vi "Example.vi"() -> ()   [LabVIEW 2015]
uses:
  BufferConfig.ctl
  BufferLogging.lvlib
panel:
  out "snapshot":sgl[][](graph)
  in  "logging trigger":bool
  in  "stop":bool
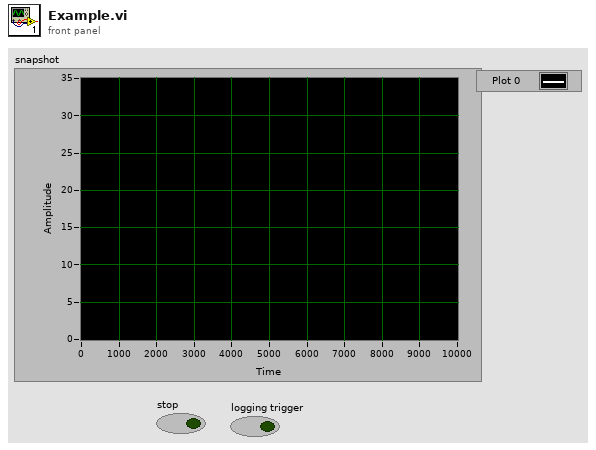
[diagram p1: front panel]
types:
  T1 = typedef "BufferLogging.lvlib/BufferConfig.ctl" = cluster{"Channels":string[], "pretriggerTime_sec":dbl, "posttriggerTime_sec":dbl, "BlockSizePerChannel":i32, "SampleRate_Hz":dbl, "decimation factor":i32, "logDirectory":path, "logPrefix":string, "max files":i32}
  T2 = typedef "BufferLogging.lvlib/Buffers.ctl" = cluster{"Channels":string[], "PosttriggerBuffer":refnum<queue>, "PretriggerBuffer":refnum<queue>, "BlockSizePerChannel":i32, " logging semaphore":T3, "Log refnum":refnum<k34>, "snapshotBuffer":refnum<data-value>, "logDirectory":path, "logPrefix":string, "decimation factor":i32, "max files":i32, "SampleRate":dbl}
  T3 = typedef "Semaphore RefNum" = refnum<k1>
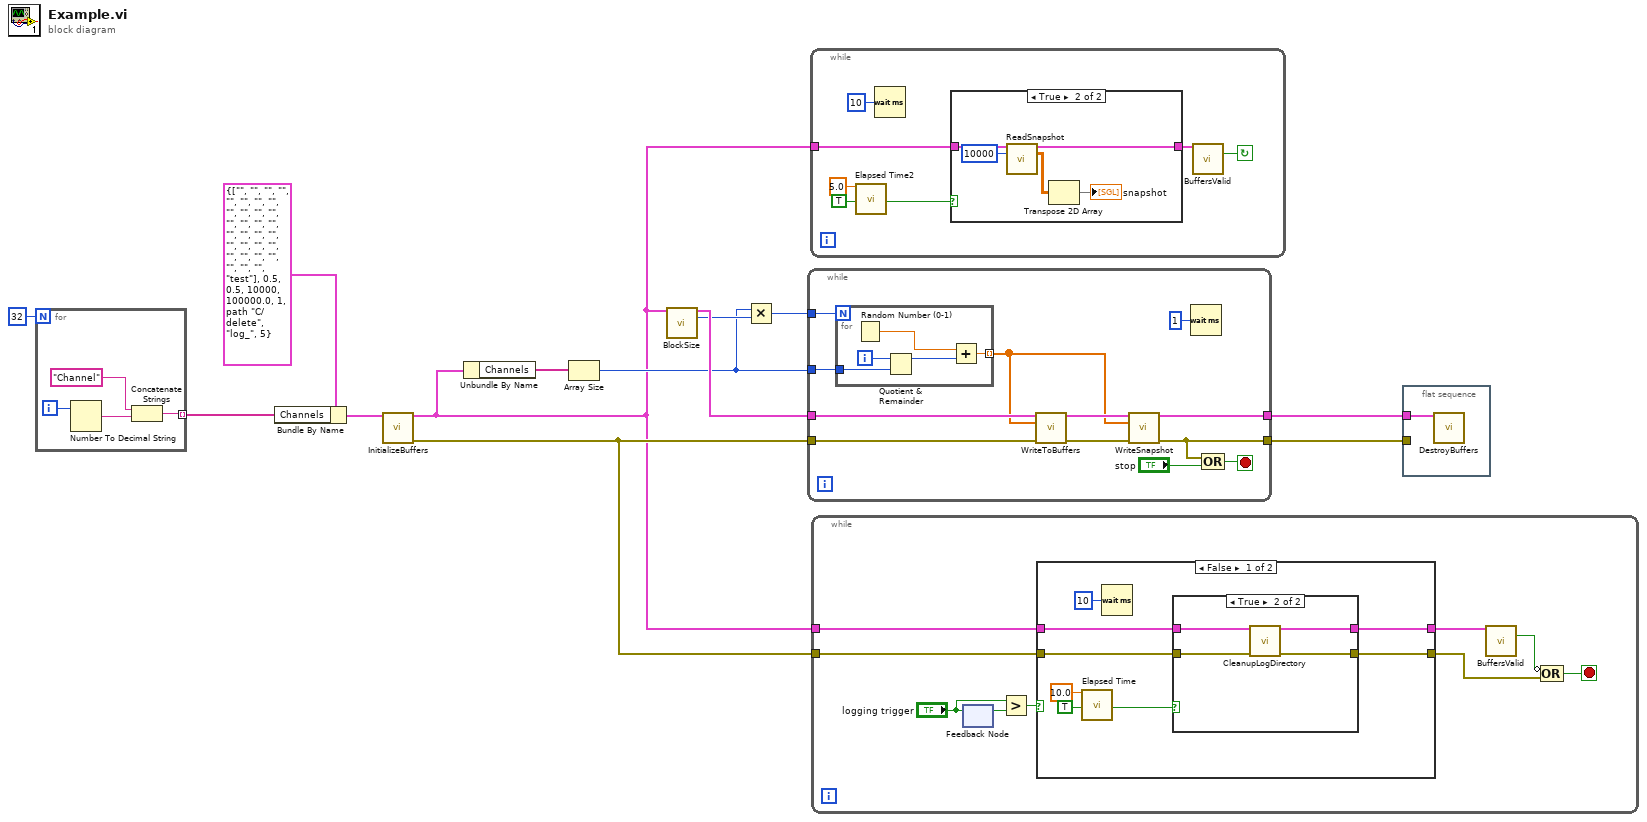
[diagram p0: block diagram]
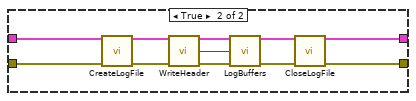
[diagram p4: hidden frame]
diagram:
  n1 = for {
    N: 32 -> [_]
    tunnel: [w14] -> w4 mode=indexing
    i -> [w17]
    n2 = Number To Decimal String(number=w17) -> (decimal integer string=w16:string)  [unwired: 1 in]
    n3 = Concatenate Strings("Channel", w16) -> (w14:string)
  }
  n4 = Bundle By Name(cluster=T1 {"Channels"=["", "", "", "", "", "", "", "", "", "", "", "", "", "", "", "", "", "", "", "", "", "", "", "", "", "", "", "", "", "", "", "test"], "pretriggerTime_sec"=0.5, "posttriggerTime_sec"=0.5, "BlockSizePerChannel"=10000, "SampleRate_Hz"=100000.0, "decimation factor"=1, "logDirectory"=path "C:/delete", "logPrefix"="log_", "max files"=5} ("BufferConfig"), "Channels"=w4) -> (w5:T1)
  n5 = call "InitializeBuffers.vi"("BufferConfig"=w5) -> ("Buffers"=w1:T2, "error out"=w3:errorcluster)  [unwired: 13 in]
  n6 = Unbundle By Name(w1) -> ("Channels"=w8:string[])
  n7 = Array Size(array=w8) -> (size(s)=w7:i32)
  n8 = call "BlockSize.vi"("BuffersIn"=w1) -> ("BuffersOut"=w12:T2, "BlockSize"=w10:i32)  [unwired: 13 in]
  n9 = Multiply(x=w7, y=w10) -> (x*y=w9:i32)
  n10 = while {
    tunnel: w12 -> [w29]
    tunnel: w3 -> [w28]
    tunnel: [w25] -> w13
    tunnel: w9 -> [w22]
    tunnel: [w20] -> w11
    tunnel: w7 -> [w18]
    stop <- w24 stop-if-true
    n11 = for {
      N: w22 -> [_]
      tunnel: [w33] -> w21 mode=indexing
      tunnel: w18 -> [w30]
      i -> [w32]
      n12 = Random Number (0-1)() -> (number: 0 to 1=w34:dbl)
      n13 = Quotient & Remainder(x=w32, y=w30) -> (x-y*floor(x/y)=w31:i32)  [unwired: 1 out]
      n14 = Add(x=w34, y=w31) -> (x+y=w33:dbl)
    }
    n15 = call "WriteToBuffers.vi"("Buffers in"=w29, "Data"=w21, "error in (no error)"=w28) -> ("Buffers out"=w27:T2, "error out"=w26:errorcluster)  [unwired: 11 in]
    n16 = call "WriteSnapshot.vi"("Buffers in"=w27, "Snapshot"=w21, "error in (no error)"=w26) -> ("Buffers out"=w25:T2, "error out"=w20:errorcluster)  [unwired: 11 in]
    n17 = Wait (ms)(milliseconds to wait=u32 1) -> ()  [unwired: 1 out]
    n18 = Compound Arithmetic op=OR(w20, "stop") -> (w24:bool)
  }
  n19 = while {
    tunnel: w1 -> [w41]
    stop <- w39 continue-if-true
    n20 = call "Elapsed Time2"("Time Target (s)"=5.0, "Auto Reset"=TRUE) -> ("Time has Elapsed"=w36:bool)  [unwired: 10 in, 7 out]
    n21 = Wait (ms)(milliseconds to wait=u32 10) -> ()  [unwired: 1 out]
    n22 = case shown="True" w36 {
      tunnel: w41 -> [w42 w47]
      tunnel: [w42 w46] -> w40
      frame False {
      }
      frame True {
        n23 = call "ReadSnapshot.vi"("Buffers in"=w47, "sizeOfBlock"=10000) -> ("Buffers out"=w46:T2, "snapshot"=w44:sgl[][])  [unwired: 11 in, 1 out]
        n24 = Transpose 2D Array(2D array=w44) -> (transposed array=→"snapshot":sgl[][])
      }
    }
    n25 = call "BuffersValid.vi"("Buffers in"=w40) -> ("valid"=w39:bool)  [unwired: 13 in, 1 out]
  }
  n26 = while {
    tunnel: w3 -> [w53]
    tunnel: w1 -> [w52]
    stop <- w50 stop-if-true
    n27 = feedback-in #1("logging trigger") -> ()
    n28 = feedback #1() -> (w55:bool)  [unwired: 1 in]
    n29 = Greater?(x="logging trigger", y=w55) -> (0:w54:bool)
    n30 = case shown="False" w54 {
      tunnel: w53 -> [w60 w81]
      tunnel: w52 -> [w58 w80]
      tunnel: [w57 w72] -> w51
      tunnel: [w59 w71] -> w48
      frame False {
        n31 = call "Elapsed Time"("Time Target (s)"=10.0, "Auto Reset"=TRUE) -> ("Time has Elapsed"=w61:bool)  [unwired: 10 in, 7 out]
        n32 = Wait (ms)(milliseconds to wait=u32 10) -> ()  [unwired: 1 out]
        n33 = case shown="True" w61 {
          tunnel: w60 -> [w66 w70]
          tunnel: [w66 w69] -> w59
          tunnel: w58 -> [w65 w68]
          tunnel: [w65 w67] -> w57
          frame False {
          }
          frame True {
            n34 = call "CleanupLogDirectory.vi"("BuffersIn"=w68, "error in"=w70) -> ("BuffersOut"=w67:T2, "error out"=w69:errorcluster)  [unwired: 12 in]
          }
        }
      }
      frame True {
        n35 = call "CreateLogFile.vi"("Buffers in"=w80, "error in (no error)"=w81) -> ("Buffers out"=w79:T2, "error out"=w78:errorcluster)  [unwired: 12 in]
        n36 = call "WriteHeader.vi"("Buffers in"=w79, "error in (no error)"=w78) -> ("Buffers out"=w77:T2, "numOfChannels"=w75:i32, "error out"=w76:errorcluster)  [unwired: 11 in]
        n37 = call "LogBuffers.vi"("Buffers in"=w77, "numOfChannels"=w75, "error in (no error)"=w76) -> ("Buffers out"=w74:T2, "error out"=w73:errorcluster)  [unwired: 11 in]
        n38 = call "CloseLogFile.vi"("Buffers in"=w74, "error in (no error)"=w73) -> ("Buffers out"=w72:T2, "error out"=w71:errorcluster)  [unwired: 11 in, 1 out]
      }
    }
    n39 = call "BuffersValid.vi"("Buffers in"=w51) -> ("valid"=w49:bool)  [unwired: 13 in, 1 out]
    n40 = Compound Arithmetic op=OR(invert w49, w48) -> (w50:bool)
  }
  n41 = flat-sequence {
    tunnel: w13 -> [w82]
    tunnel: w11 -> [_]
    frame #0 {
      n42 = call "DestroyBuffers.vi"("Buffers"=w82) -> ()  [unwired: 14 in, 1 out]
    }
  }
